vi "Debouncer_HasElapsed.vi"(8 "CurrentTIme":dbl=-1.0, 11 "Debouncer In":T1 {"PrevTimeSeconds" format="%13.6p"; "DebounceTimeSeconds" format="%13.6p"}) -> (0 "CurrentTimeOut":dbl format="%33.4f", 3 "HasElapsed":bool)   [LabVIEW 2019, in "Trajectory_Library.lvlib"]
doc: "Internal function\n\nSee if debounce time has elapsed."
uses:
  Trajectory_Library.lvlib
  DEBOUNCER.ctl
  DEBOUNCER_TYPE_ENUM.ctl
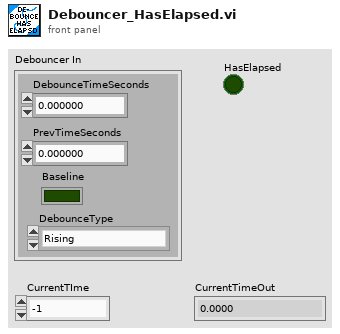
[diagram p1: front panel]
types:
  T1 = typedef "Trajectory_Library.lvlib/DEBOUNCER.ctl" = cluster{"DebounceTimeSeconds":dbl, "PrevTimeSeconds":dbl, "Baseline":bool, "DebounceType":T2}
  T2 = typedef "Trajectory_Library.lvlib/DEBOUNCER_TYPE_ENUM.ctl" = enum16{"Rising", "Falling", "Both"}
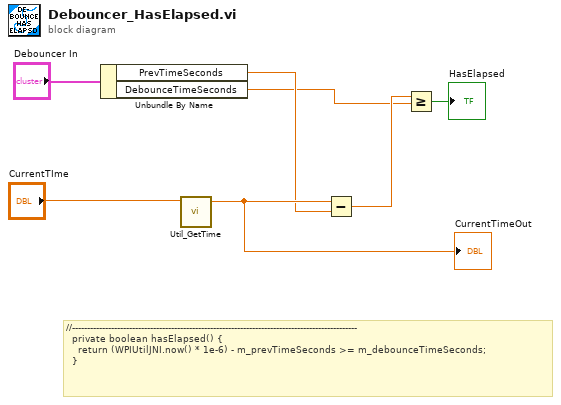
[diagram p0: block diagram]
diagram:
  # "//-----------------------------------------------------------------------------------------------\n  private boolean hasElapsed() {\n    return (WPIUtilJNI.now() * 1e-6) - m_prevTimeSeconds >= m_debounceTimeSeconds;\n  }"
  n1 = Unbundle By Name("Debouncer In") -> ("PrevTimeSeconds"=w4:dbl, "DebounceTimeSeconds"=w2:dbl)
  n2 = call "Util_GetTime.vi"("Pass_Through_Time"="CurrentTIme") -> ("FPGA_Time_Seconds"=w5:dbl)  [unwired: 9 in, 1 out]
  "CurrentTimeOut" <- w5
  n3 = Subtract(x=w5, y=w4) -> (x-y=w3:dbl)
  n4 = Greater Or Equal?(x=w3, y=w2) -> (x >= y?=→"HasElapsed":bool)
